vi "test_simple_Doppler_filtered.vi"() -> ()   [LabVIEW 2009]
doc: "Copyright (C) 2009, Stepan A. Baranov\nweb: http://www.OCTLab.org/\nemail: stepan@baranov.su"
uses:
  OCTLib.dll
panel:
  out "error out":errorcluster
  out "max":dbl
  out "min":dbl
  out "width":i32
  out "height":i32
  in  "Small/Big":bool
  out "loop #":i32
  out "RSM_STAT time":u32
  out "LabView time":u32
  out "RSM_STAT Array":dbl[][](array[numeric])
  out "LabView Array":dbl[][](array[numeric])
  in  "stop":bool
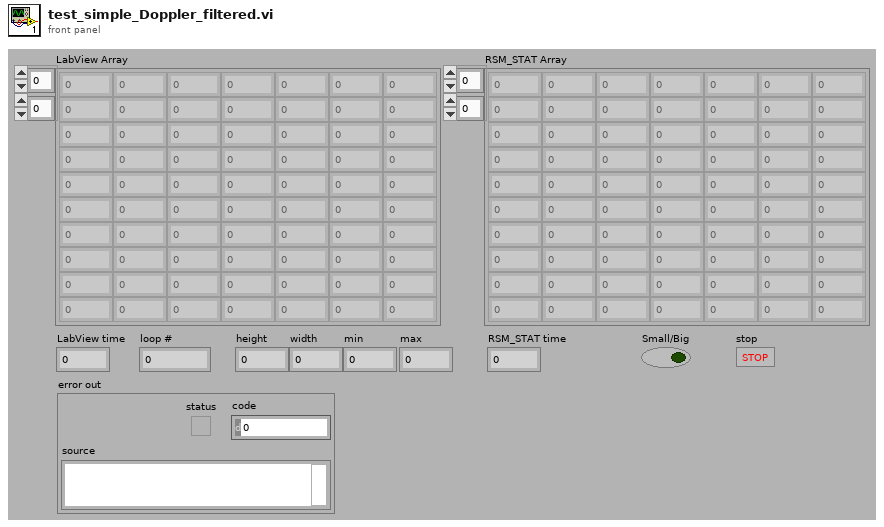
[diagram p1: front panel]
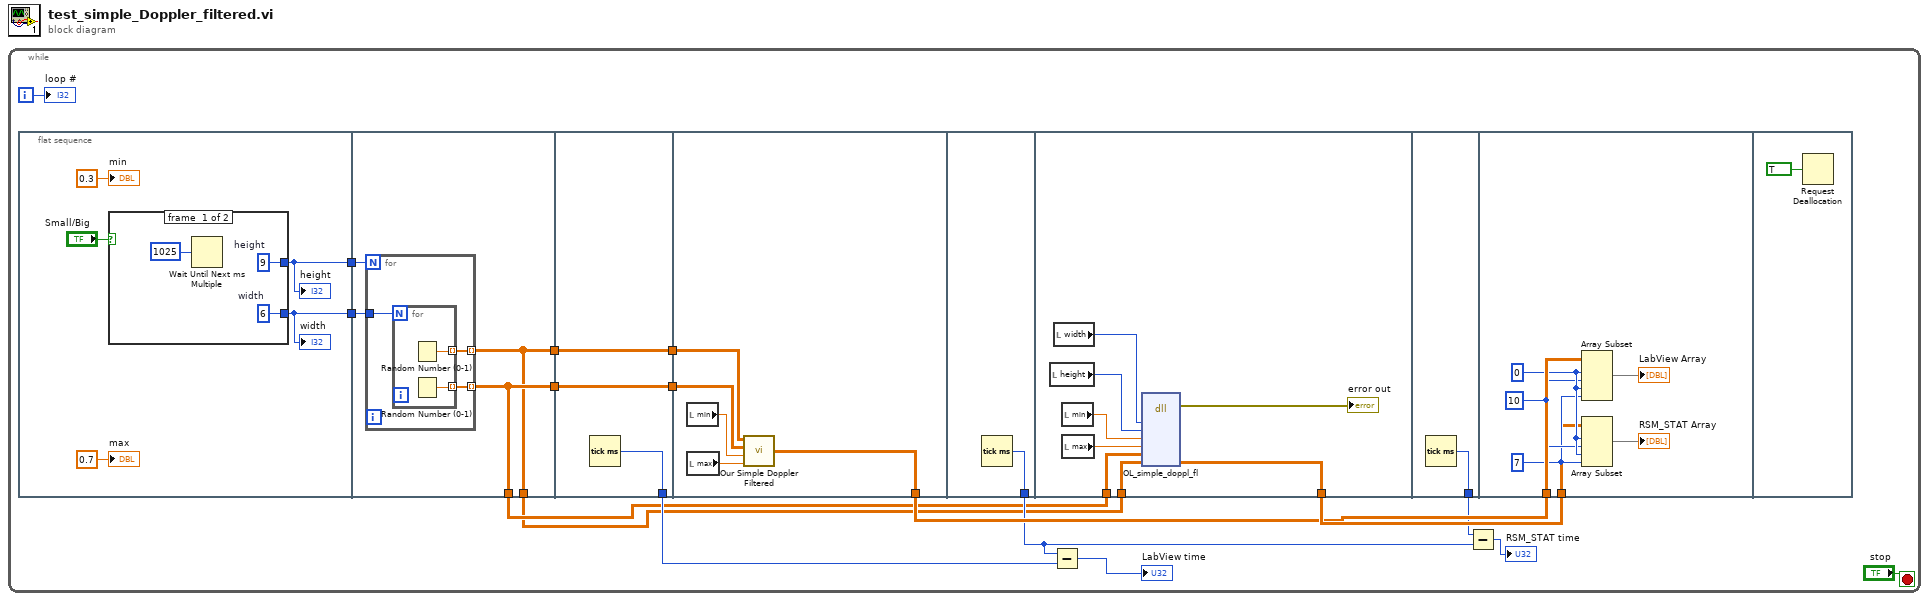
[diagram p0: block diagram]
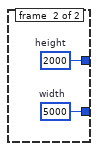
[diagram p2: hidden frame]
diagram:
  n1 = while {
    i -> [w9]
    stop <- "stop" stop-if-true
    n2 = flat-sequence {
      tunnel: [w21] -> w5
      tunnel: [w20] -> w4
      tunnel: [w29] -> w8
      tunnel: [w29] -> w6
      tunnel: w5 -> [w31]
      tunnel: w4 -> [w30]
      tunnel: [w28] -> w3
      tunnel: [w28] -> w1
      tunnel: [w39] -> w14
      tunnel: [w38] -> w7
      tunnel: w6 -> [w38]
      tunnel: w3 -> [w37]
      tunnel: [w37] -> w2
      tunnel: [w40] -> w15
      tunnel: w7 -> [w43]
      tunnel: w2 -> [w44]
      tunnel: [w45] -> w11
      tunnel: w8 -> [w48]
      tunnel: [w51] -> w16
      tunnel: w1 -> [w47]
      tunnel: [w54] -> w12
      tunnel: w16 -> [w55]
      tunnel: w15 -> [w61]
      frame #0 {
        n3 = case shown="True" "Small/Big" {
          tunnel: [w24 w27] -> w20
          tunnel: [w25 w26] -> w21
          frame #0 {
            w25 = 6  # width
            w24 = 9  # height
            n4 = Wait Until Next ms Multiple(millisecond multiple=u32 1025) -> ()  [unwired: 1 out]
          }
          frame #1 {
            w26 = 5000  # width
            w27 = 2000  # height
          }
        }
        "height" <- w20
        "width" <- w21
        "min" <- 0.3 ("min")
        "max" <- 0.7 ("max")
      }
      frame #1 {
        n5 = for {
          N: w30 -> [_]
          tunnel: w31 -> [w34]
          tunnel: [w33] -> w29 mode=indexing
          tunnel: [w32] -> w28 mode=indexing
          n6 = for {
            N: w34 -> [_]
            tunnel: [w36] -> w33 mode=indexing
            tunnel: [w35] -> w32 mode=indexing
            n7 = Random Number (0-1)() -> (number: 0 to 1=w35:dbl)
            n8 = Random Number (0-1)() -> (number: 0 to 1=w36:dbl)
          }
        }
      }
      frame #2 {
        n9 = Tick Count (ms)() -> (millisecond timer value=w39:u32)
      }
      frame #3 {
        n10 = local read "min"() -> (w42:dbl)
        n11 = local read "max"() -> (w41:dbl)
        n12 = call "Our Simple Doppler Filtered.vi"("max"=w41, "min"=w42, "intensity"=w43, "phase"=w44) -> ("2D Doppler Image"=w40:dbl[][])
      }
      frame #4 {
        n13 = Tick Count (ms)() -> (millisecond timer value=w45:u32)
      }
      frame #5 {
        n14 = local read "height"() -> (w52:i32)
        n15 = local read "width"() -> (w53:i32)
        n16 = local read "min"() -> (w50:dbl)
        n17 = local read "max"() -> (w49:dbl)
        n18 = dll-call lib="OCTLib.dll" fn="OL_simple_doppl_fl"("width"=w53, "height"=w52, "min"=w50, "max"=w49, "ref"=w48, "data"=w47) -> (error out=→"error out":errorcluster, "data"=w51:dbl[][])  [unwired: 9 in, 1 out]
      }
      frame #6 {
        n19 = Tick Count (ms)() -> (millisecond timer value=w54:u32)
      }
      frame #7 {
        w58 = 10 ("length")
        w57 = 7 ("length")
        w59 = 0 ("index")
        n20 = Array Subset(array=w61, index (row)=w59, length (row)=w58, index (col)=w59, length (col)=w57) -> (→"LabView Array":dbl[][])
        n21 = Array Subset(array=w55, index (row)=w59, length (row)=w58, index (col)=w59, length (col)=w57) -> (→"RSM_STAT Array":dbl[][])
      }
      frame #8 {
        n22 = Request Deallocation(TRUE ("flag")) -> ()
      }
    }
    n23 = Subtract(x=w11, y=w14) -> (x-y=→"LabView time":u32)
    n24 = Subtract(x=w12, y=w11) -> (x-y=→"RSM_STAT time":u32)
    "loop #" <- w9
  }
